vi "TestAsterMove.vi"() -> ()   [LabVIEW 2017]
uses:
  ManageMovableObjects/ManRef_mods.ctl
  Display/Display_mods.ctl
  Asteroid/Asteroid_data.ctl
  GameConfig/GameConfig_data.ctl
  <userlib>/_OpenG.lib/numeric/numeric.llb/Random Number Within Range - DBL__ogtk.vi
  <userlib>/_OpenG.lib/numeric/numeric.llb/Random Number Within Range - I32__ogtk.vi
panel:
  out "error out":errorcluster
  in  "Add":bool
  in  "stop":bool
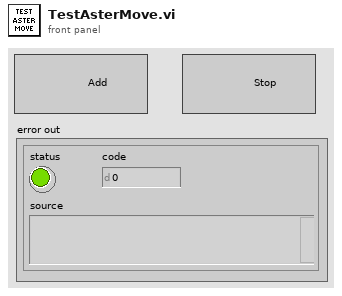
[diagram p1: front panel]
types:
  T1 = typedef "GameConfig_data.ctl" = cluster{"SpaceShip":cluster{"Angle":dbl, "SideLenght":dbl, "MaxLinearVeloc":dbl, "MaxAngularVeloc":dbl, "LinearAceleration":dbl, "AngularAceleration":dbl}, "Physics":cluster{"LinearDragFactor":dbl, "AngularDragFactor":dbl}, "Asteroids":cluster{"MaxSize":dbl, "MaxDivisions":i32, "MaxVeloc":dbl, "MinVeloc":dbl, "Fill":bool}, "Environment":cluster{"MaxAsteroids":i32, "TimeIncrement":dbl, "AsterProbCreation":dbl}, "Shots":cluster{"MinTimeShots":dbl, "ShotSize":dbl, "ShotSpeed":dbl}}
  T2 = typedef "Display_mods.ctl" = enum16{"Init", "GetBase", "DrawAster", "DrawShip", "DrawShoot", "Clear", "Close"}
  T3 = typedef "ManRef_mods.ctl" = enum16{"Init", "NewAster", "MoveAll", "DestroyAster", "NewShoot", "DestroyShot", "CheckColision", "End"}
  T4 = typedef "Asteroid_data.ctl" = cluster{"Veloc":dbl, "Direction":dbl, "Size":i32, "displayRef":refnum<vi>, "Max X":dbl, "Max Y":dbl, "Xpos":dbl, "Ypos":dbl, "ID":i32, "Config":T1}
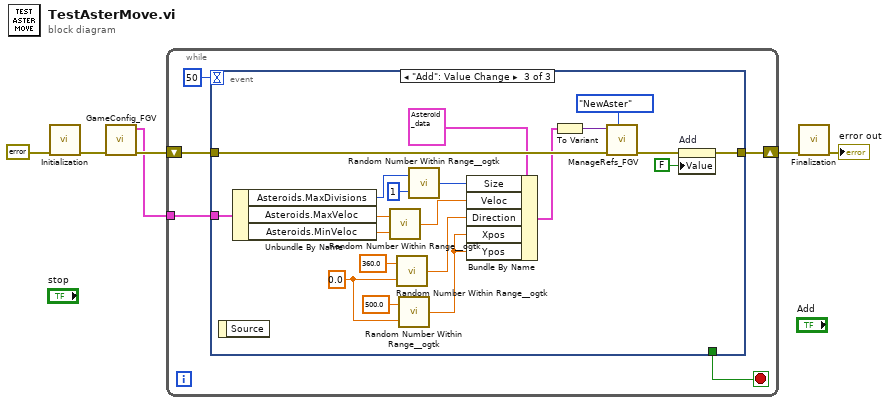
[diagram p0: block diagram]
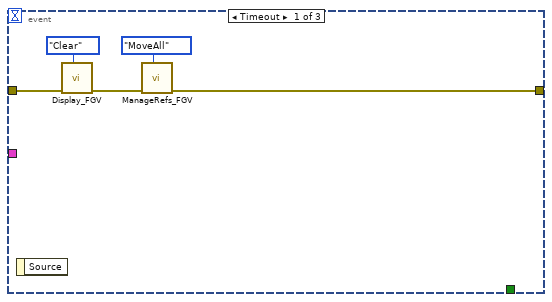
[diagram p2: hidden frame]
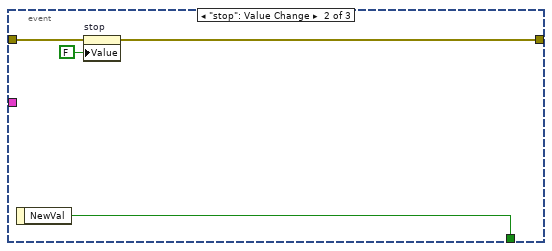
[diagram p3: hidden frame]
diagram:
  n1 = call "Initialization.vi"("error in"=errorcluster {"status"=FALSE, "code"=0, "source"=""}) -> ("error out"=w3:errorcluster)  [unwired: 10 in]
  n2 = call "GameConfig_FGV.vi"("error in"=w3) -> ("error out"=w2:errorcluster, "Config"=w1:T1)  [unwired: 9 in]
  n3 = while {
    shift-right: [w10] -> w5
    shift-left: w2 -> [w11]
    tunnel: w1 -> [w7]
    stop <- w8 stop-if-true
    n4 = event shown="[2] \"Add\": Value Change" {
      selector: _ -> [_ _ _]
      dyn-events: _ -> [_ _ _]
      timeout: 50 -> [_ _ _]
      tunnel: w11 -> [w13 w18 w40]
      tunnel: [w15 w17 w37] -> w10
      tunnel: [_ w20 _] -> w8
      tunnel: w7 -> [_ _ w35]
      event Timeout {
        n5 = event-data() -> ()  [unwired: 1 in, 1 out]
        n6 = call "Display_FGV.vi"("Display_mods"=Display_mods."Clear", "error in"=w13) -> ("error out"=w12:errorcluster)  [unwired: 8 in, 1 out]
        n7 = call "ManageRefs_FGV.vi"("ManRef_mods"=ManRef_mods."MoveAll", "error in"=w12) -> ("error out"=w15:errorcluster)  [unwired: 9 in]
      }
      event "stop": Value Change {
        n8 = event-data() -> ("NewVal"=w20:bool)  [unwired: 1 in]
        n9 = property on="stop" class="Bool (strict)"(error in=w18, "Value"=FALSE ("Add")) -> (error out=w17:errorcluster)  [unwired: 1 in, 1 out]
      }
      event "Add": Value Change {
        w23 = 0.0 ("Low")
        n10 = event-data() -> ()  [unwired: 1 in, 1 out]
        n11 = Unbundle By Name(w35) -> ("Asteroids.MaxDivisions"=w32:i32, "Asteroids.MaxVeloc"=w34:dbl, "Asteroids.MinVeloc"=w33:dbl)
        n12 = call-poly <userlib>:"Random Number Within Range__ogtk.vi"("High"=w34, "Low"=w33) -> ("Random Number"=w28:dbl)  [unwired: 3 in]
        n13 = call-poly <userlib>:"Random Number Within Range__ogtk.vi"("High"=360.0, "Low"=w23) -> ("Random Number"=w27:dbl)  [unwired: 3 in]
        n14 = call-poly <userlib>:"Random Number Within Range__ogtk.vi"("High"=500.0, "Low"=w23) -> ("Random Number"=w25:dbl)  [unwired: 3 in]
        n15 = call-poly <userlib>:"Random Number Within Range__ogtk.vi"("High"=w32, "Low"=1) -> ("Random Number"=w29:i32)  [unwired: 3 in]
        n16 = Bundle By Name(cluster=T4 {"Veloc"=100.0, "Direction"=0.0, "Size"=3, "displayRef"=refnum, "Max X"=0.0, "Max Y"=0.0, "Xpos"=0.0, "Ypos"=150.0, "ID"=0, "Config"={"SpaceShip"={"Angle"=30.0, "SideLenght"=2.0, "MaxLinearVeloc"=10.0, "MaxAngularVeloc"=10.0, "LinearAceleration"=1.0, "AngularAceleration"=1.0}, "Physics"={"LinearDragFactor"=1.0, "AngularDragFactor"=1.0}, "Asteroids"={"MaxSize"=6.0, "MaxDivisions"=3, "MaxVeloc"=8.0, "MinVeloc"=1.0, "Fill"=FALSE}, "Environment"={"MaxAsteroids"=10, "TimeIncrement"=0.1, "AsterProbCreation"=0.1}, "Shots"={"MinTimeShots"=10.0, "ShotSize"=0.1, "ShotSpeed"=0.1}}} ("AsteroidData"), "Size"=w29, "Veloc"=w28, "Direction"=w27, "Xpos"=w25, "Ypos"=w25) -> (w24:T4)
        n17 = To Variant(anything=w24) -> (Variant=w39:variant)
        n18 = call "ManageRefs_FGV.vi"("ManRef_mods"=ManRef_mods."NewAster", "error in"=w40, "DataIn"=w39) -> ("error out"=w38:errorcluster)  [unwired: 8 in]
        n19 = property on="Add" class="Bool (strict)"(error in=w38, "Value"=FALSE ("Add")) -> (error out=w37:errorcluster)  [unwired: 1 in, 1 out]
      }
    }
  }
  n20 = call "Finalization.vi"("error in"=w5) -> ("error out"=→"error out":errorcluster)  [unwired: 10 in]
